vi "Delete HTML&PDFnames.vi"(8 "error in (no error)":errorcluster, 11 "Folder_Mgmt":refnum<class "Folder_Mgmt.lvclass">) -> (0 "error out":errorcluster, 3 "Folder_Mgmt 2":refnum<class "Folder_Mgmt.lvclass">)   [LabVIEW 2016, in "Folder_Mgmt.lvclass"]
doc: "This VI deletes a DVR reference variable."
uses:
  Folder_Mgmt.lvclass
  Folder_Mgmt.lvclass/Folder_Mgmt.ctl
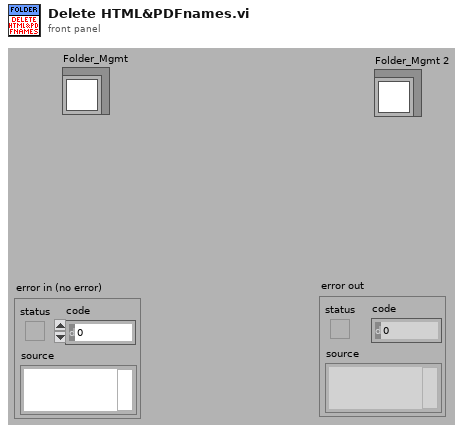
[diagram p1: front panel]
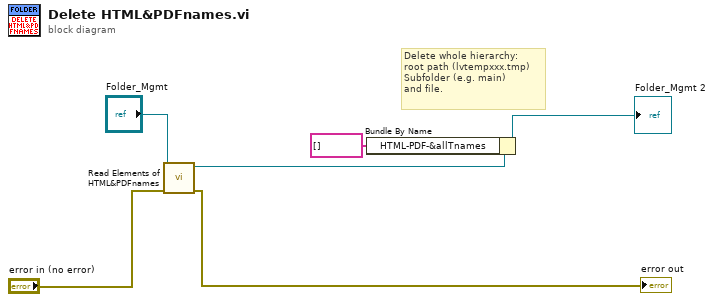
[diagram p0: block diagram]
diagram:
  # "Delete whole hierarchy:\nroot path (lvtempxxx.tmp)\nSubfolder (e.g. main)\nand file."
  n1 = call "Read Elements of HTML&PDFnames.vi"("error in (no error)"="error in (no error)", "Folder_Mgmt"="Folder_Mgmt") -> ("error out"=→"error out":errorcluster, "Folder_Mgmt 2"=w1:refnum<class "Folder_Mgmt.lvclass">)  [unwired: 7 in, 1 out]
  n2 = Bundle By Name(cluster=w1, "HTML-PDF-&allTnames"=string[] [] ("PDFnames")) -> (→"Folder_Mgmt 2":refnum<class "Folder_Mgmt.lvclass">)
